vi "DBTableName-Log.vi"() -> (1 "DB Table Name":string)   [LabVIEW 2015, in "MainController.lvlib"]
uses:
  MainController.lvlib
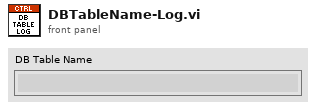
[diagram p1: front panel]
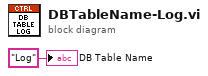
[diagram p0: block diagram]
diagram:
  "DB Table Name" <- "Log" ("ProcessName")
